vi "Wolna na wysw FVG.vi"(7 "Akcja (GET)":T1, 8 "error in (no error)":errorcluster, 11 "Wolna in":T2) -> (0 "error out":errorcluster, 3 "Wolna out":T2)   [LabVIEW 2013]
doc: "Use this template to build a VI to use as a subVI."
uses:
  Kontrolki/Przetwarzanie/Kanaly.ctl
  Kontrolki/FVGs/FVG akcje podstawowa.ctl
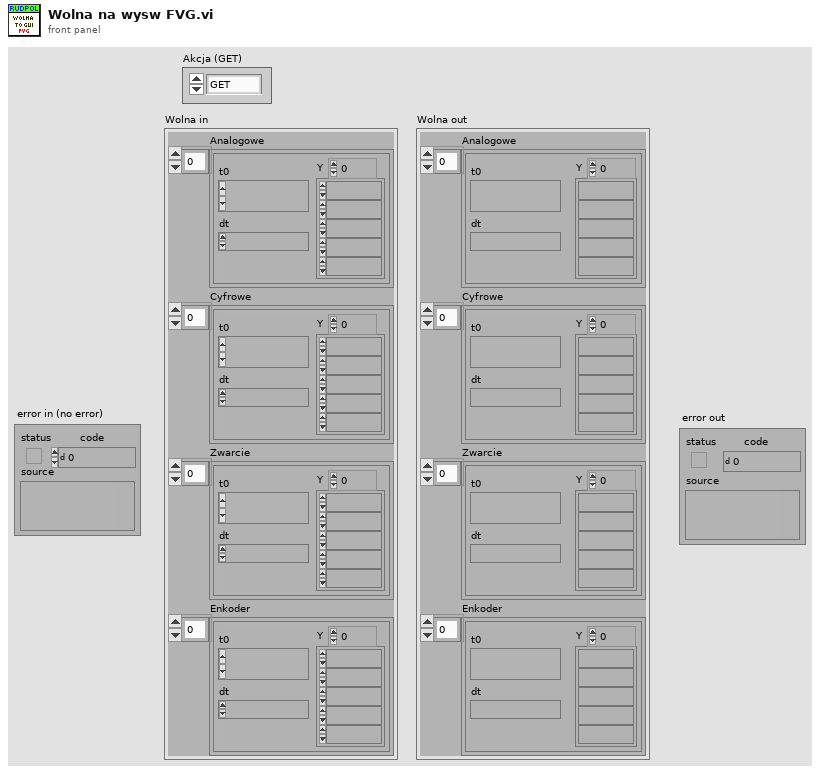
[diagram p1: front panel]
types:
  T1 = typedef "FVG akcje podstawowa.ctl" = enum16{"GET", "SET"}
  T2 = typedef "Kanaly.ctl" = cluster{"Analogowe":waveform(dbl)[], "Cyfrowe":waveform(dbl)[], "Zwarcie":waveform(dbl)[], "Enkoder":waveform(dbl)[]}
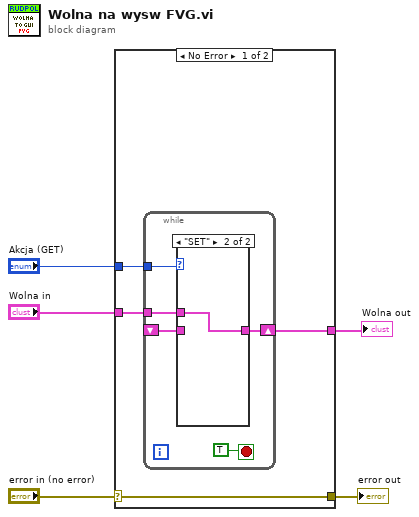
[diagram p0: block diagram]
diagram:
  n1 = case shown="No Error" "error in (no error)" {
    selector: "error in (no error)" -> [w9 w18]
    tunnel: [w9 w18] -> w4
    tunnel: "Wolna in" -> [w8 w17]
    tunnel: [w7 w17] -> w2
    tunnel: "Akcja (GET)" -> [w6 _]
    frame No Error {
      n2 = while {
        tunnel: w8 -> [w13]
        shift-right: [w12] -> w7
        shift-left: _ -> [w11]
        tunnel: w6 -> [w10]
        stop <- TRUE stop-if-true
        n3 = case shown="\"SET\"" w10 {
          tunnel: w13 -> [_ w16]
          tunnel: [w15 w16] -> w12
          tunnel: w11 -> [w15 _]
          frame "GET", Default {
          }
          frame "SET" {
          }
        }
      }
    }
    frame Error {
    }
  }
  "error out" <- w4
  "Wolna out" <- w2
